vi "Autonomous Independent.vi"() -> ()   [LabVIEW 2016]
doc: "This VI is called when autonomous begins, and will automatically be terminated when autonomous ends. You can carry out timed or sensor driven robot movement independently without needing to return to the caller."
uses:
  2_8_17/Auto_Action.ctl
  <vilib>/Rock Robotics/Network Tables/NT Read Number.vi
  2_11_17/Systems/Global 1.vi
panel:
  out "Auto Mode":dbl=10.0
  in  "Auton_Modes":T2(array[cluster])=[{"Actions"=[{"Effort"=0.55, "Duration"=3.5, "Action"=enum."Nothing", "Encoder"=0.0, "Condition"=FALSE}, {"Effort"=0.0, "Duration"=0.0, "Action"=enum."Nothing", "Encoder"=0.0, "Condition"=FALSE}]}, {"Actions"=[{"Effort"=0.53, "Duration"=1.0, "Action"=enum."Shoot", "Encoder"=6.462, "Condition"=TRUE}, {"Effort"=0.0, "Duration"=3.0, "Action"=enum."Index", "Encoder"=0.0, "Condition"=FALSE}, {"Effort"=0.3, "Duration"=2.0, "Action"=enum."Turn", "Encoder"=38.0, "Condition"=FALSE}, {"Effort"=0.3, "Duration"=5.0, "Action"=enum."Drive", "Encoder"=0.0, "Condition"=TRUE}, {"Effort"=0.25, "Duration"=0.0, "Action"=enum."Nothing", "Encoder"=57.0, "Condition"=FALSE}, {"Effort"=-0.25, "Duration"=0.0, "Action"=enum."Nothing", "Encoder"=0.0, "Condition"=FALSE}, {"Effort"=1.0, "Duration"=0.0, "Action"=enum."Nothing", "Encoder"=0.0, "Condition"=FALSE}, {"Effort"=0.25, "Duration"=0.0, "Action"=enum."Nothing", "Encoder"=0.0, "Condition"=FALSE}]}, {"Actions"=[{"Effort"=0.0, "Duration"=0.1, "Action"=enum."Drive Encoder Reset", "Encoder"=0.0, "Condition"=FALSE}, {"Effort"=0.0, "Duration"=1.0, "Action"=enum."Gyro Reset", "Encoder"=0.0, "Condition"=FALSE}, {"Effort"=0.3, "Duration"=2.5, "Action"=enum."Drive", "Encoder"=1000.0, "Condition"=TRUE}, {"Effort"=1.0, "Duration"=1.0, "Action"=enum."Gear0", "Encoder"=0.0, "Condition"=FALSE}, {"Effort"=1.0, "Duration"=0.0, "Action"=enum."Nothing", "Encoder"=0.0, "Condition"=FALSE}, {"Effort"=1.0, "Duration"=0.5, "Action"=enum."Nothing", "Encoder"=0.0, "Condition"=FALSE}, {"Effort"=0.0, "Duration"=0.0, "Action"=enum."Drive Encoder Reset", "Encoder"=0.0, "Condition"=FALSE}, {"Effort"=0.3, "Duration"=0.5, "Action"=enum."Nothing", "Encoder"=24.0, "Condition"=TRUE}, {"Effort"=0.0, "Duration"=0.0, "Action"=enum."Nothing", "Encoder"=0.0, "Condition"=FALSE}, {"Effort"=-0.2, "Duration"=2.0, "Action"=enum."Drive", "Encoder"=24.0, "Condition"=TRUE}, {"Effort"=0.0, "Duration"=0.0, "Action"=enum."Drive Encoder Reset", "Encoder"=0.0, "Condition"=FALSE}, {"Effort"=-0.25, "Duration"=0.0, "Action"=enum."Nothing", "Encoder"=12.0, "Condition"=FALSE}]}, {"Actions"=[{"Effort"=0.0, "Duration"=0.1, "Action"=enum."Drive Encoder Reset", "Encoder"=6.462, "Condition"=FALSE}, {"Effort"=0.0, "Duration"=0.1, "Action"=enum."Gyro Reset", "Encoder"=0.0, "Condition"=FALSE}, {"Effort"=-0.25, "Duration"=1.0, "Action"=enum."Drive", "Encoder"=6.462, "Condition"=FALSE}, {"Effort"=0.0, "Duration"=0.1, "Action"=enum."Gyro Reset", "Encoder"=0.0, "Condition"=FALSE}, {"Effort"=-0.25, "Duration"=0.0, "Action"=enum."Turn", "Encoder"=0.0, "Condition"=FALSE}, {"Effort"=-0.25, "Duration"=0.0, "Action"=enum."Drive", "Encoder"=7.5, "Condition"=FALSE}, {"Effort"=-1.0, "Duration"=0.0, "Action"=enum."Gear0", "Encoder"=0.0, "Condition"=FALSE}, {"Effort"=0.25, "Duration"=0.0, "Action"=enum."Drive", "Encoder"=3.0, "Condition"=FALSE}]}, {"Actions"=[{"Effort"=0.0, "Duration"=0.1, "Action"=enum."Drive Encoder Reset", "Encoder"=6.462, "Condition"=FALSE}, {"Effort"=0.0, "Duration"=0.1, "Action"=enum."Gyro Reset", "Encoder"=0.0, "Condition"=FALSE}, {"Effort"=-0.25, "Duration"=1.0, "Action"=enum."Drive", "Encoder"=6.462, "Condition"=FALSE}, {"Effort"=0.0, "Duration"=0.1, "Action"=enum."Gyro Reset", "Encoder"=0.0, "Condition"=FALSE}, {"Effort"=-0.25, "Duration"=0.0, "Action"=enum."Turn", "Encoder"=0.0, "Condition"=FALSE}, {"Effort"=-0.25, "Duration"=0.0, "Action"=enum."Drive", "Encoder"=7.5, "Condition"=FALSE}, {"Effort"=-1.0, "Duration"=0.0, "Action"=enum."Gear0", "Encoder"=0.0, "Condition"=FALSE}, {"Effort"=0.25, "Duration"=0.0, "Action"=enum."Drive", "Encoder"=3.0, "Condition"=FALSE}]}, {"Actions"=[{"Effort"=0.0, "Duration"=0.1, "Action"=enum."Drive Encoder Reset", "Encoder"=0.0, "Condition"=FALSE}, {"Effort"=0.0, "Duration"=0.1, "Action"=enum."Gyro Reset", "Encoder"=0.0, "Condition"=FALSE}, {"Effort"=0.25, "Duration"=1.0, "Action"=enum."Drive", "Encoder"=6.462, "Condition"=FALSE}, {"Effort"=1.0, "Duration"=0.1, "Action"=enum."Gyro Reset", "Encoder"=0.0, "Condition"=FALSE}, {"Effort"=0.25, "Duration"=0.0, "Action"=enum."Turn", "Encoder"=0.0, "Condition"=FALSE}, {"Effort"=0.25, "Duration"=0.0, "Action"=enum."Drive", "Encoder"=7.5, "Condition"=FALSE}, {"Effort"=1.0, "Duration"=0.0, "Action"=enum."Gear0", "Encoder"=0.0, "Condition"=FALSE}, {"Effort"=-0.25, "Duration"=0.0, "Action"=enum."Drive", "Encoder"=3.0, "Condition"=FALSE}]}, {"Actions"=[{"Effort"=0.0, "Duration"=0.1, "Action"=enum."Nothing", "Encoder"=0.0, "Condition"=FALSE}, {"Effort"=0.0, "Duration"=0.1, "Action"=enum."Gyro Reset", "Encoder"=0.0, "Condition"=FALSE}, {"Effort"=0.25, "Duration"=5.0, "Action"=enum."Drive", "Encoder"=60000.0, "Condition"=TRUE}, {"Effort"=0.75, "Duration"=1.0, "Action"=enum."Nothing", "Encoder"=0.0, "Condition"=FALSE}, {"Effort"=0.0, "Duration"=1.0, "Action"=enum."Nothing", "Encoder"=0.0, "Condition"=FALSE}, {"Effort"=0.0, "Duration"=0.0, "Action"=enum."Nothing", "Encoder"=0.0, "Condition"=FALSE}]}, {"Actions"=[{"Effort"=0.0, "Duration"=0.5, "Action"=enum."Drive Encoder Reset", "Encoder"=0.0, "Condition"=FALSE}, {"Effort"=0.55, "Duration"=4.25, "Action"=enum."Gyro Reset", "Encoder"=0.0, "Condition"=FALSE}, {"Effort"=-0.5, "Duration"=0.0, "Action"=enum."Drive", "Encoder"=46.0, "Condition"=FALSE}, {"Effort"=0.3, "Duration"=1.0, "Action"=enum."Nothing", "Encoder"=0.0, "Condition"=FALSE}, {"Effort"=0.3, "Duration"=2.0, "Action"=enum."Vision Correction", "Encoder"=76.6, "Condition"=FALSE}, {"Effort"=-0.25, "Duration"=1.0, "Action"=enum."Drive", "Encoder"=18.5, "Condition"=TRUE}, {"Effort"=1.0, "Duration"=0.0, "Action"=enum."Gear0", "Encoder"=0.0, "Condition"=FALSE}, {"Effort"=0.3, "Duration"=1.3, "Action"=enum."Drive", "Encoder"=30.0, "Condition"=TRUE}, {"Effort"=0.0, "Duration"=0.0, "Action"=enum."Nothing", "Encoder"=0.0, "Condition"=FALSE}, {"Effort"=0.03, "Duration"=0.0, "Action"=enum."Turn", "Encoder"=0.0, "Condition"=FALSE}, {"Effort"=0.0, "Duration"=0.0, "Action"=enum."Drive", "Encoder"=0.0, "Condition"=FALSE}]}, {"Actions"=[{"Effort"=0.0, "Duration"=0.0, "Action"=enum."Nothing", "Encoder"=0.0, "Condition"=FALSE}]}, {"Actions"=[{"Effort"=0.0, "Duration"=2.5, "Action"=enum."Shoot", "Encoder"=0.0, "Condition"=FALSE}, {"Effort"=0.0, "Duration"=5.0, "Action"=enum."Index", "Encoder"=0.0, "Condition"=FALSE}, {"Effort"=0.25, "Duration"=3.5, "Action"=enum."Nothing", "Encoder"=88.0, "Condition"=FALSE}, {"Effort"=1.0, "Duration"=1.0, "Action"=enum."Nothing", "Encoder"=0.0, "Condition"=FALSE}, {"Effort"=1.0, "Duration"=1.0, "Action"=enum."Nothing", "Encoder"=0.0, "Condition"=FALSE}, {"Effort"=1.0, "Duration"=0.5, "Action"=enum."Nothing", "Encoder"=0.0, "Condition"=FALSE}, {"Effort"=0.0, "Duration"=0.0, "Action"=enum."Nothing", "Encoder"=0.0, "Condition"=FALSE}, {"Effort"=-0.25, "Duration"=0.0, "Action"=enum."Nothing", "Encoder"=3.0, "Condition"=FALSE}, {"Effort"=0.0, "Duration"=0.0, "Action"=enum."Nothing", "Encoder"=0.0, "Condition"=FALSE}, {"Effort"=0.25, "Duration"=0.0, "Action"=enum."Nothing", "Encoder"=24.0, "Condition"=FALSE}, {"Effort"=0.0, "Duration"=0.0, "Action"=enum."Nothing", "Encoder"=0.0, "Condition"=FALSE}, {"Effort"=-0.25, "Duration"=0.0, "Action"=enum."Nothing", "Encoder"=12.0, "Condition"=FALSE}]}, {"Actions"=[{"Effort"=0.0, "Duration"=0.1, "Action"=enum."Drive Encoder Reset", "Encoder"=0.0, "Condition"=FALSE}, {"Effort"=0.0, "Duration"=1.0, "Action"=enum."Gyro Reset", "Encoder"=0.0, "Condition"=FALSE}, {"Effort"=0.3, "Duration"=1.4, "Action"=enum."Drive", "Encoder"=88.0, "Condition"=TRUE}, {"Effort"=0.3, "Duration"=4.0, "Action"=enum."Turn", "Encoder"=2.0, "Condition"=TRUE}, {"Effort"=1.0, "Duration"=1.0, "Action"=enum."Nothing", "Encoder"=0.0, "Condition"=FALSE}, {"Effort"=1.0, "Duration"=0.5, "Action"=enum."Nothing", "Encoder"=0.0, "Condition"=FALSE}, {"Effort"=0.0, "Duration"=0.0, "Action"=enum."Nothing", "Encoder"=0.0, "Condition"=FALSE}, {"Effort"=-0.25, "Duration"=0.0, "Action"=enum."Nothing", "Encoder"=3.0, "Condition"=FALSE}, {"Effort"=0.0, "Duration"=0.0, "Action"=enum."Nothing", "Encoder"=0.0, "Condition"=FALSE}, {"Effort"=0.25, "Duration"=0.0, "Action"=enum."Nothing", "Encoder"=24.0, "Condition"=FALSE}, {"Effort"=0.0, "Duration"=0.0, "Action"=enum."Nothing", "Encoder"=0.0, "Condition"=FALSE}, {"Effort"=-0.25, "Duration"=0.0, "Action"=enum."Nothing", "Encoder"=12.0, "Condition"=FALSE}]}, {"Actions"=[{"Effort"=0.0, "Duration"=1.0, "Action"=enum."Drive Encoder Reset", "Encoder"=0.0, "Condition"=FALSE}, {"Effort"=0.0, "Duration"=1.0, "Action"=enum."Shoot", "Encoder"=0.0, "Condition"=FALSE}, {"Effort"=0.25, "Duration"=5.0, "Action"=enum."Index", "Encoder"=88.0, "Condition"=FALSE}, {"Effort"=1.0, "Duration"=1.0, "Action"=enum."Nothing", "Encoder"=0.0, "Condition"=FALSE}, {"Effort"=1.0, "Duration"=1.0, "Action"=enum."Nothing", "Encoder"=0.0, "Condition"=FALSE}, {"Effort"=1.0, "Duration"=0.5, "Action"=enum."Nothing", "Encoder"=0.0, "Condition"=FALSE}, {"Effort"=0.0, "Duration"=0.0, "Action"=enum."Nothing", "Encoder"=0.0, "Condition"=FALSE}, {"Effort"=-0.25, "Duration"=0.0, "Action"=enum."Nothing", "Encoder"=3.0, "Condition"=FALSE}, {"Effort"=0.0, "Duration"=0.0, "Action"=enum."Nothing", "Encoder"=0.0, "Condition"=FALSE}, {"Effort"=0.25, "Duration"=0.0, "Action"=enum."Nothing", "Encoder"=24.0, "Condition"=FALSE}, {"Effort"=0.0, "Duration"=0.0, "Action"=enum."Nothing", "Encoder"=0.0, "Condition"=FALSE}, {"Effort"=-0.25, "Duration"=0.0, "Action"=enum."Nothing", "Encoder"=12.0, "Condition"=FALSE}]}, {"Actions"=[{"Effort"=0.0, "Duration"=0.1, "Action"=enum."Drive Encoder Reset", "Encoder"=0.0, "Condition"=FALSE}, {"Effort"=0.0, "Duration"=1.0, "Action"=enum."Gyro Reset", "Encoder"=0.0, "Condition"=FALSE}, {"Effort"=0.3, "Duration"=1.4, "Action"=enum."Drive", "Encoder"=88.0, "Condition"=TRUE}, {"Effort"=0.3, "Duration"=4.0, "Action"=enum."Turn", "Encoder"=0.0, "Condition"=TRUE}, {"Effort"=1.0, "Duration"=1.0, "Action"=enum."Nothing", "Encoder"=0.0, "Condition"=FALSE}, {"Effort"=1.0, "Duration"=0.5, "Action"=enum."Nothing", "Encoder"=0.0, "Condition"=FALSE}, {"Effort"=0.0, "Duration"=0.0, "Action"=enum."Nothing", "Encoder"=0.0, "Condition"=FALSE}, {"Effort"=0.3, "Duration"=0.5, "Action"=enum."Nothing", "Encoder"=24.0, "Condition"=TRUE}, {"Effort"=0.0, "Duration"=0.0, "Action"=enum."Nothing", "Encoder"=0.0, "Condition"=FALSE}, {"Effort"=-0.2, "Duration"=2.0, "Action"=enum."Nothing", "Encoder"=24.0, "Condition"=TRUE}, {"Effort"=0.0, "Duration"=0.0, "Action"=enum."Nothing", "Encoder"=0.0, "Condition"=FALSE}, {"Effort"=-0.25, "Duration"=0.0, "Action"=enum."Nothing", "Encoder"=12.0, "Condition"=FALSE}]}]
  # "Nothing"
  # "Boiler Right Right side gear"
  # "Middle Gear"
  # "Boiler Right Left Side Gear"
  # "Boiler Left RightSide Gear"
  # "Boiler Left Left Side Gear"
  # "Drive"
  # "Vision Correction"
  # "Hopper"
  # "10 ball"
  # "Farside"
  # "Boilerside-10 ball"
  # "Auto 5"
  # "Auto 6"
  # "Auto 6"
  # "Auto 7"
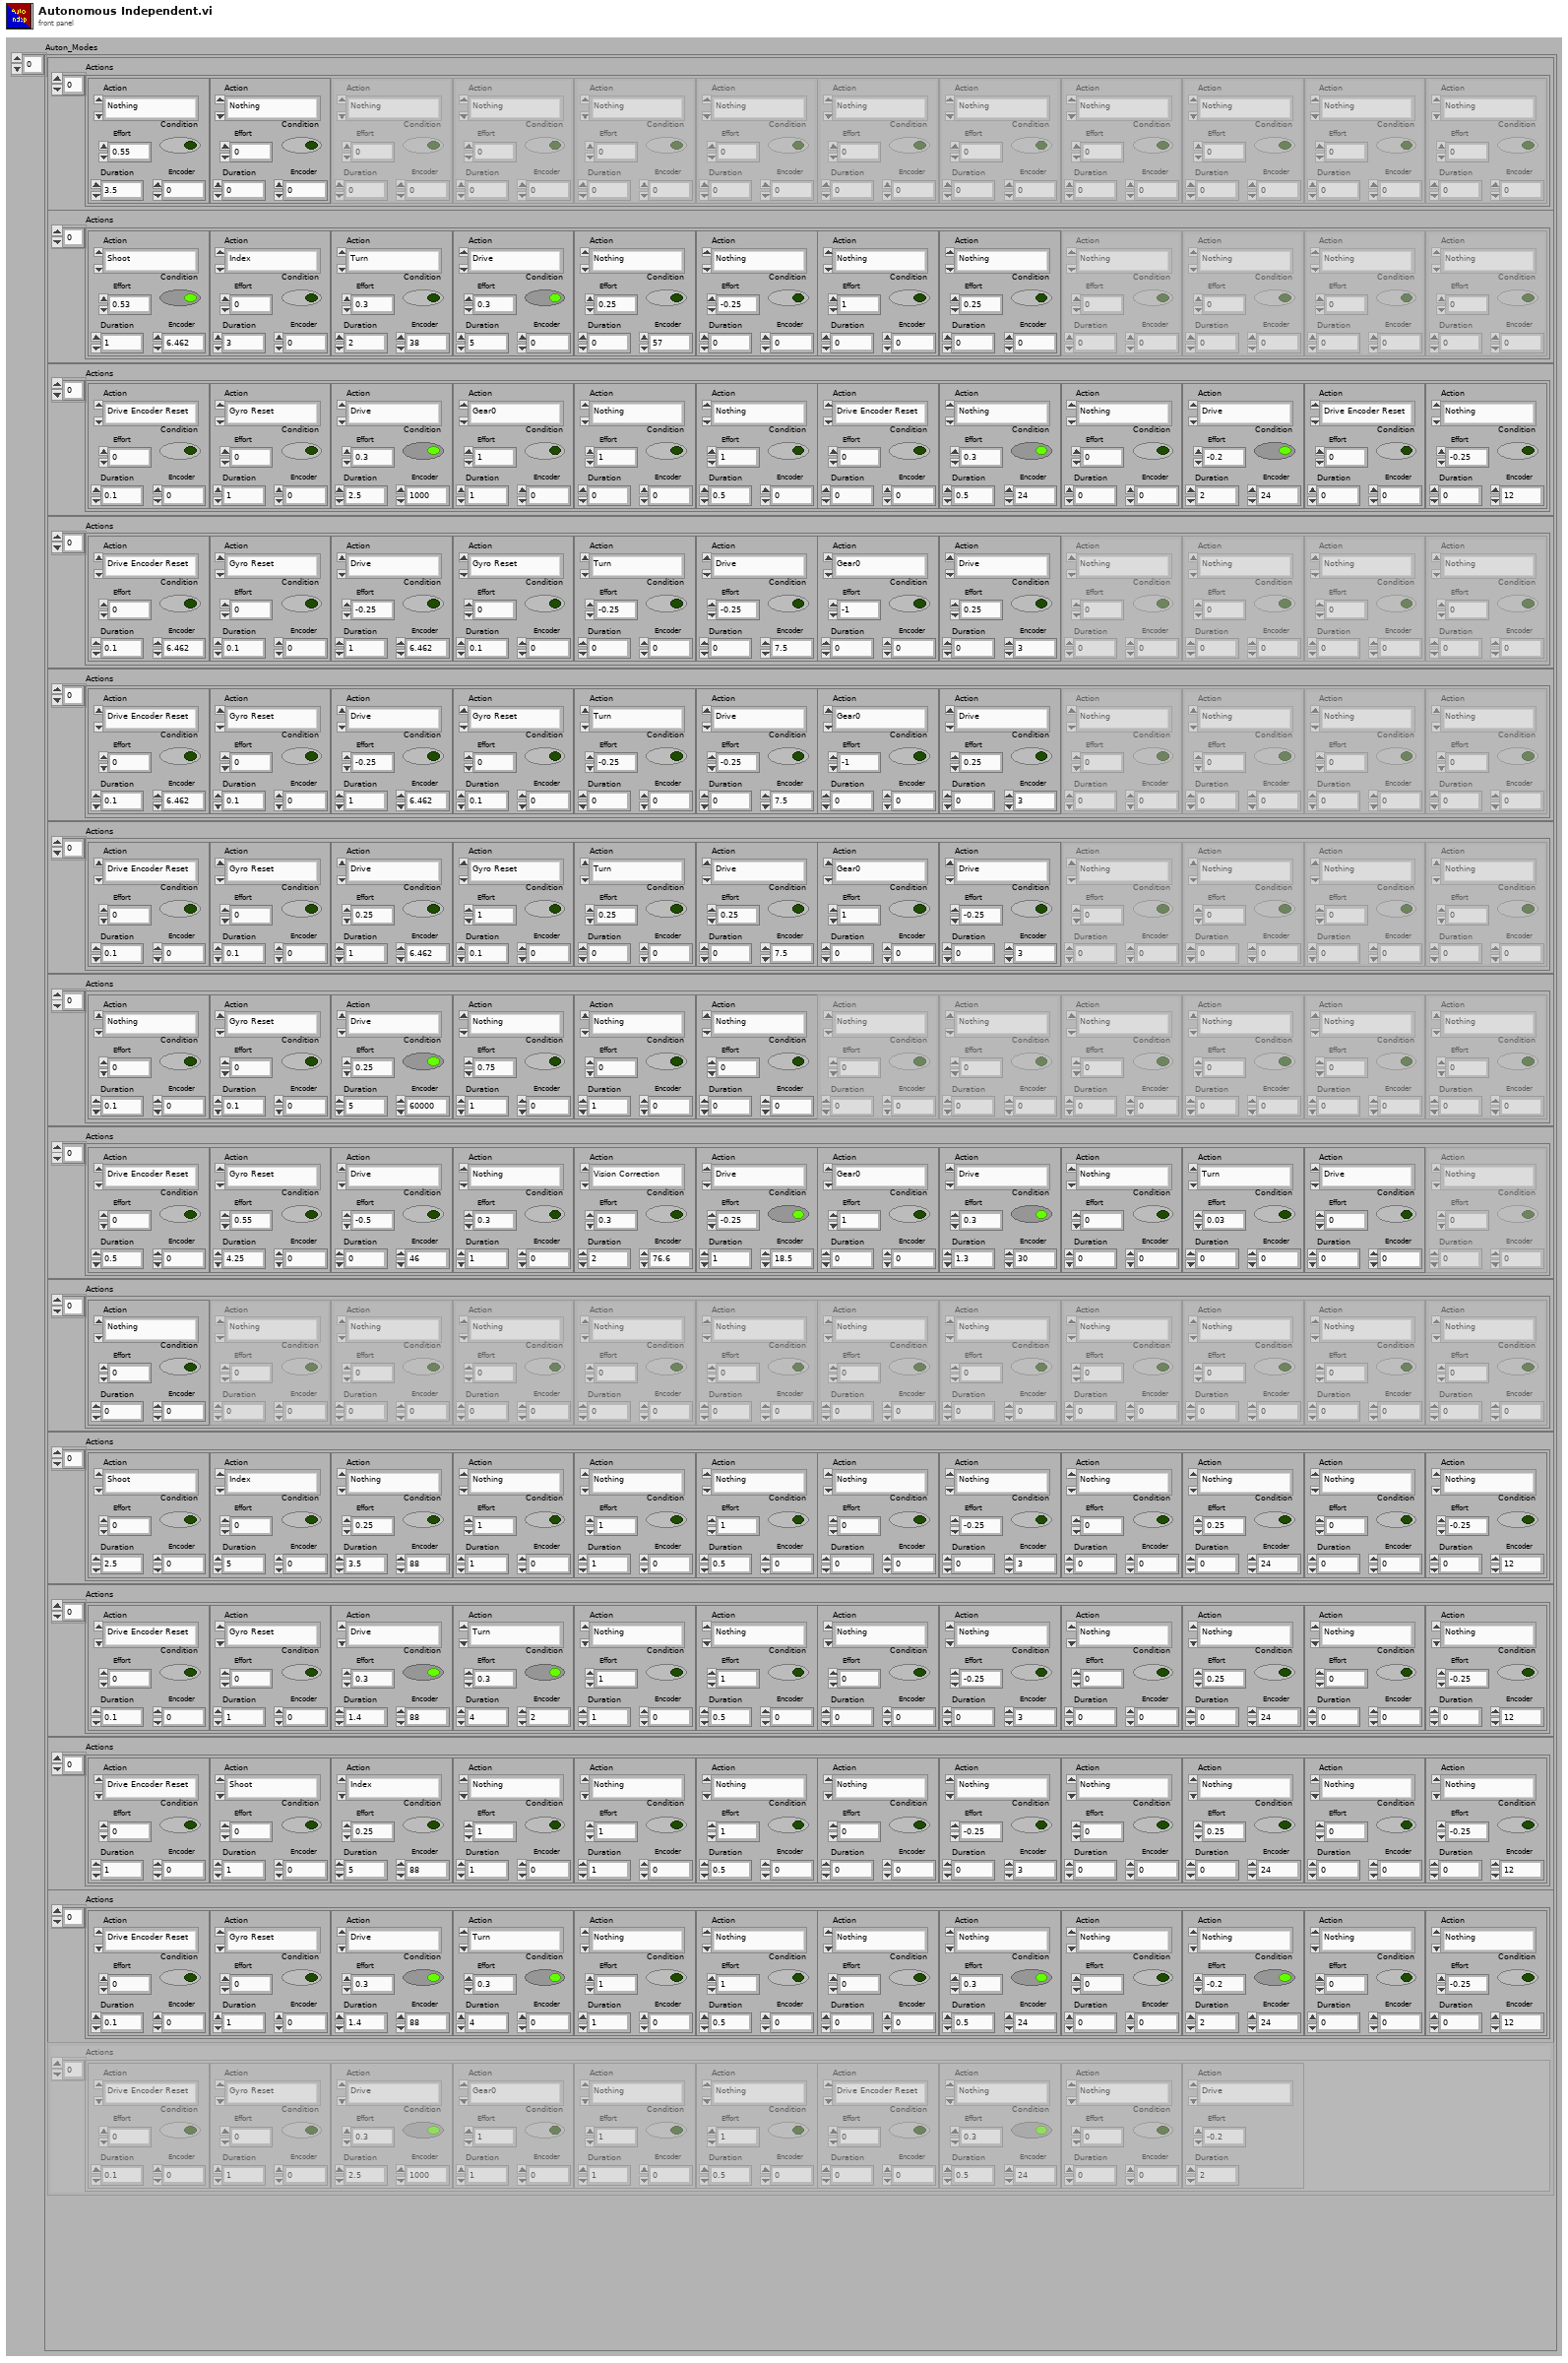
[diagram p1: front panel]
types:
  T1 = typedef "Auto_Action.ctl" = enum16{"Nothing", "Drive", "Vision Correction", "Turn", "Gear0", "Gear1", "Climb", "Intake", "Index", "Shoot", "Test", "Drive Encoder Reset", "Gyro Reset"}
  T2 = cluster{"Actions":cluster{"Effort":dbl, "Duration":dbl, "Action":T1, "Encoder":dbl, "Condition":bool}[]}[]
  T3 = cluster{"Actions":cluster{"Effort":dbl, "Duration":dbl, "Action":T1, "Encoder":dbl, "Condition":bool}[]}
  T4 = cluster{"Effort":dbl, "Duration":dbl, "Action":T1, "Encoder":dbl, "Condition":bool}[]
  T5 = typedef "WPI_MotorControlDeviceRef.ctl" = cluster{"DeviceStatus":errorcluster, "Type":T6, "PWM":cluster{"PWM Channel":T7, "DeadBand":T8}, "CAN":cluster{"Device Number":u8, "SetOutput VI Ref":variant, "GetOutput VI Ref":variant, "Enable VI Ref":variant, "Disable VI Ref":variant, "Data":variant}, "Invert":bool}
  T6 = typedef "WPI_MotorControlType.ctl" = enum16{"PWM", "CAN"}
  T7 = typedef "FPGA_DIOPWMChannel.ctl" = enum8{"PWM 0", "PWM 1", "PWM 2", "PWM 3", "PWM 4", "PWM 5", "PWM 6", "PWM 7", "PWM 8", "PWM 9", "PWM MXP 0", "PWM MXP 1", "PWM MXP 2", "PWM MXP 3", "PWM MXP 4", "PWM MXP 5", "PWM MXP 6", "PWM MXP 7", "PWM MXP 8", "PWM MXP 9", "Invalid"}
  T8 = typedef "WPI_PWMDeadband.ctl" = cluster{"Name":string, "maxPositivePwm":i32, "minPositivePwm":i32, "centerPwm":i32, "maxNegativePwm":i32, "minNegativePwm":i32, "angularRange":u16}
  T9 = typedef "WPI_CANTalonSRX_GlobalStatus.ctl" = cluster{"Applied Throttle":dbl, "Module Enabled":bool, "CAN Error":errorcluster, "Closed Loop Error":dbl, "Forward Limit Switch Closed":bool, "Reverse Limit Switch Closed":bool, "Sensor Position":dbl, "Sensor Velocity":dbl, "Current":dbl, "Sticky Fault - Over Temp":bool, "Sticky Fault - Under Voltage":bool, "Sticky Fault - Forward Limit":bool, "Sticky Fault - Reverse Limit":bool, "Sticky Fault - Forward Soft Limit":bool, "Sticky Fault - Reverse Soft Limit":bool, "Brake is Enabled":bool, "Encoder Position":dbl, "Encoder Velocity":dbl, "Encoder Index Count":dbl, "Encoder A Pin State":bool, "Encoder B Pin State":bool, "Encoder Index Pin State":bool, "Analog In":dbl, "Analog In Velocity":dbl, "Temperature (C)":dbl, "Battery Voltage":dbl, "Control 5 Is Supported":bool, "Current Profile Slot Select":dbl, "Pos Div 8":bool, "Vel Div 4":bool, "Pulse Width Position":i32, "Pulse Width Velocity":i32, "Pulse Width Rise To Rise (us)":i32, "Pulse Width Rise To Fall (us)":i32, "Mot Prof Active Is Under Run":bool, "Mot Prof Active Has Under Run":bool, "Mot Prof Active Is Last":bool, "Mot Prof Active Velocity Only":bool, "Mot Prof Active Is Valid":bool, "Mot Prof Buffer Is Full":bool, "Mot Prof Active Profile Slot Select":i32, "Mot Prof NextID":i32, "Mot Prof Count":i32, "Mot Prof Active Velocity":dbl, "Mot Prof Active Position":dbl, "Mot Prof Output Enable":i32}
  T10 = typedef "WPI_GyroDevRef.ctl" = cluster{"DevStatus":errorcluster, "Analog Channel":T11, "Offset":dbl, "Gain (VoltsPerDegree/Second)":dbl, "Gyro Type":enum16{"Analog", "XRS450"}, "Handle":i32, "SPI Bus":T12, "Device Found":bool, "Sample Rate":dbl, "Calibrate On Open":bool}
  T11 = typedef "FPGA_AIChannel.ctl" = enum8{"AI 0", "AI 1", "AI 2", "AI 3", "AI MXP 0", "AI MXP 1", "AI MXP 2", "AI MXP 3", "Invalid"}
  T12 = typedef "spi_bus.ctl" = enum16{"SPI On-Board, CS0", "SPI On-Board, CS1", "SPI On-Board, CS2", "SPI On-Board, CS3", "SPI MXP", "Invalid"}
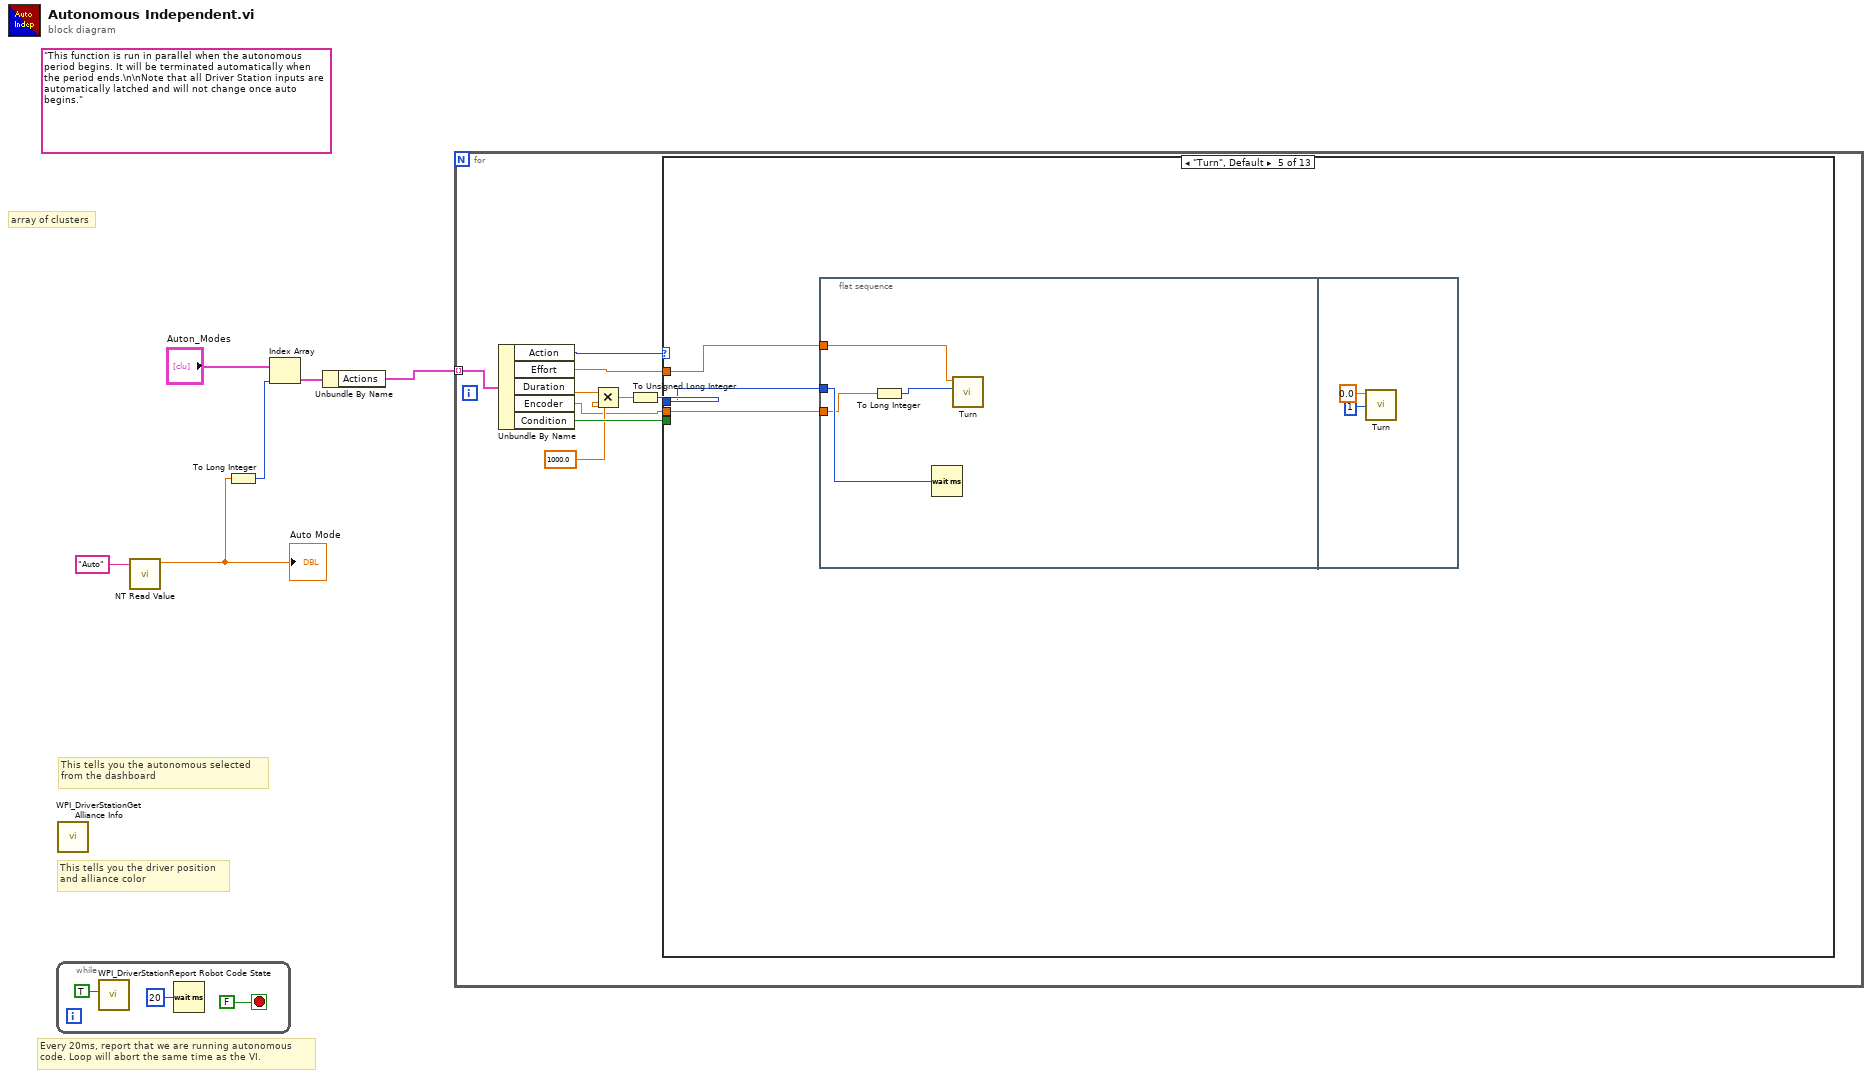
[diagram p0: block diagram]
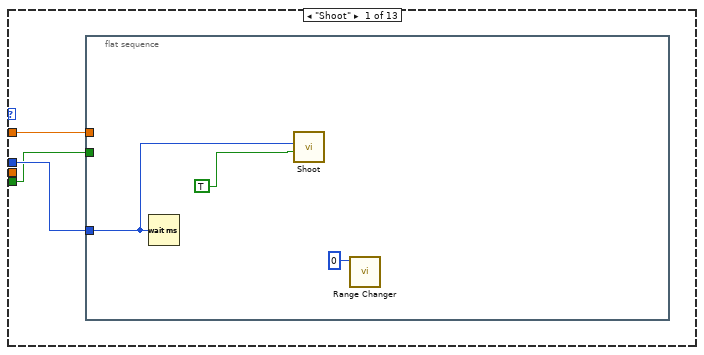
[diagram p2: hidden frame]
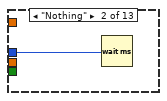
[diagram p3: hidden frame]
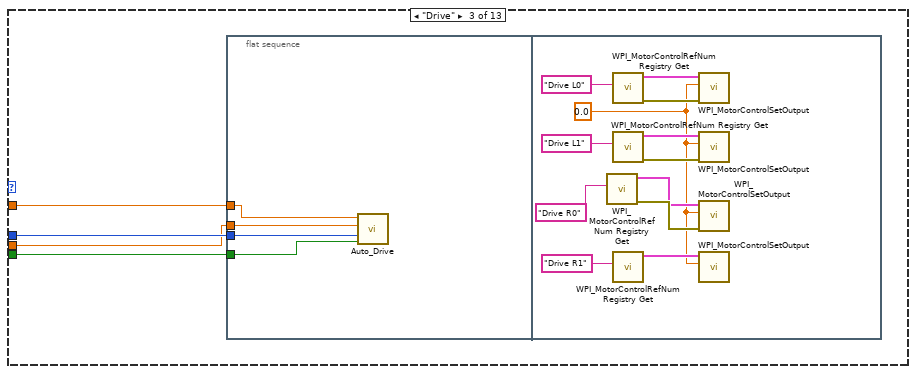
[diagram p4: hidden frame]
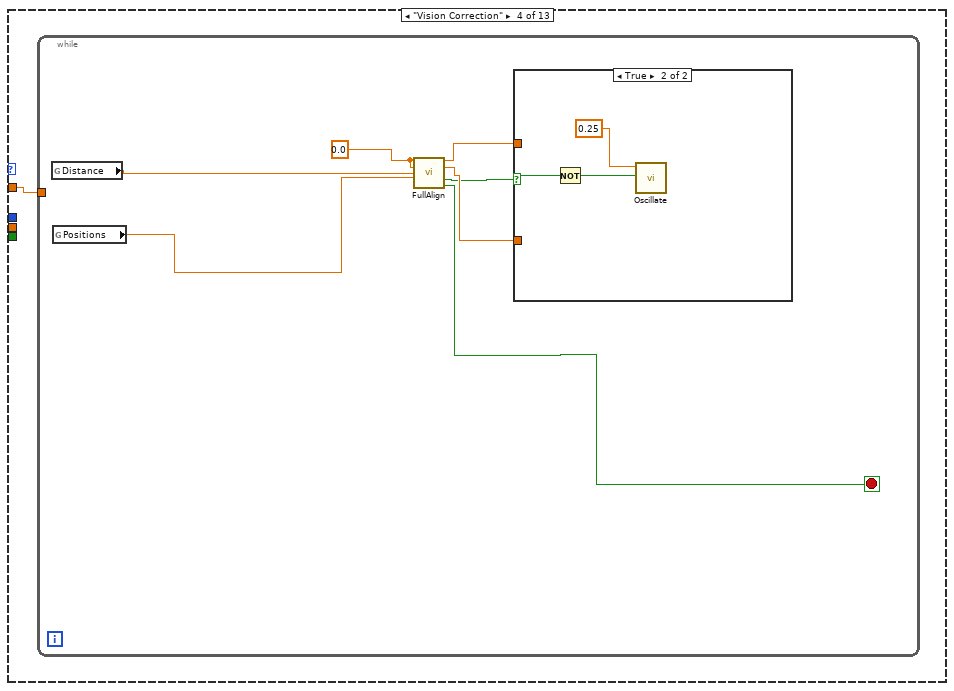
[diagram p5: hidden frame]
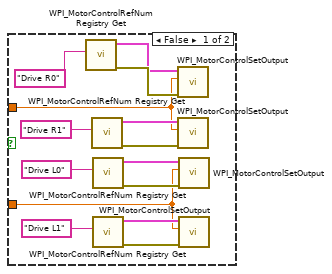
[diagram p6: hidden frame]
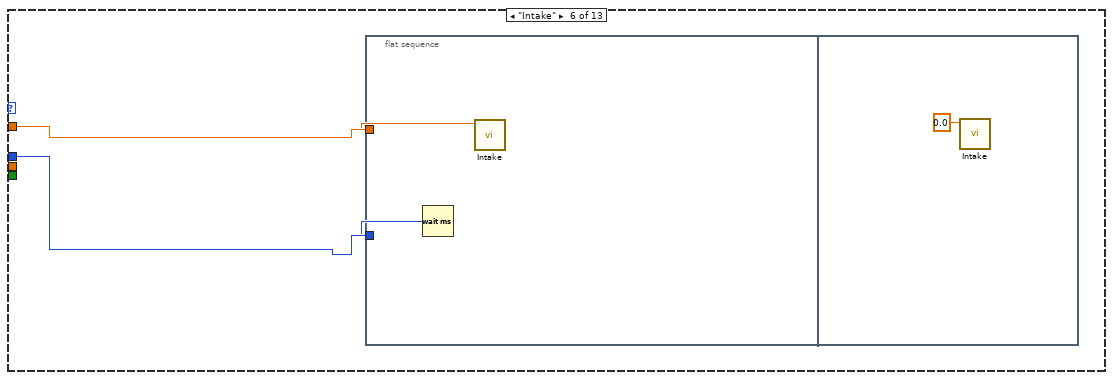
[diagram p7: hidden frame]
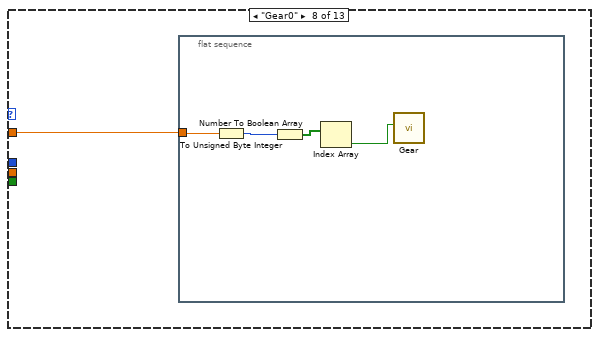
[diagram p9: hidden frame]
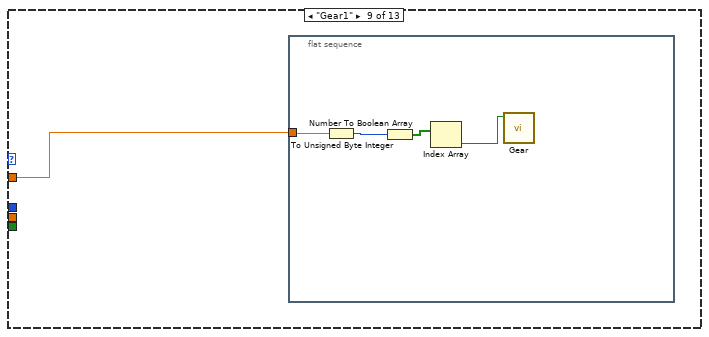
[diagram p10: hidden frame]
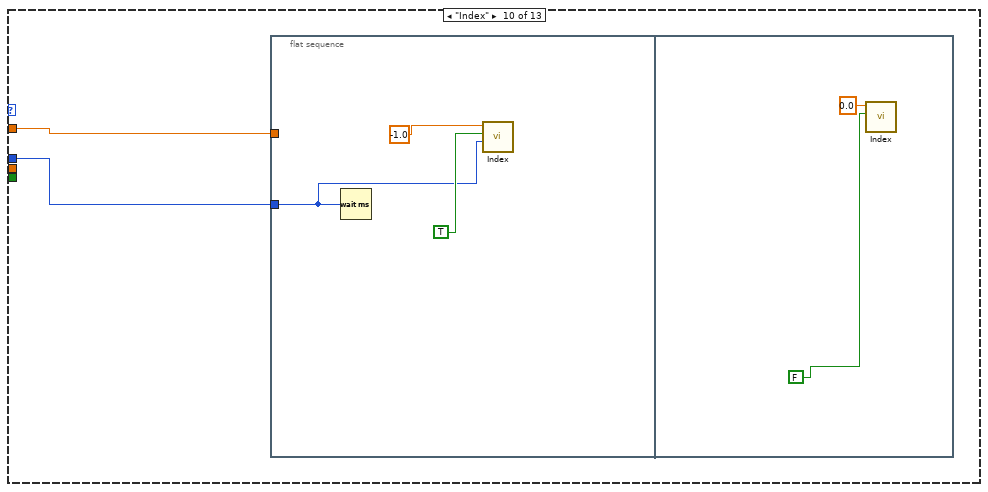
[diagram p11: hidden frame]
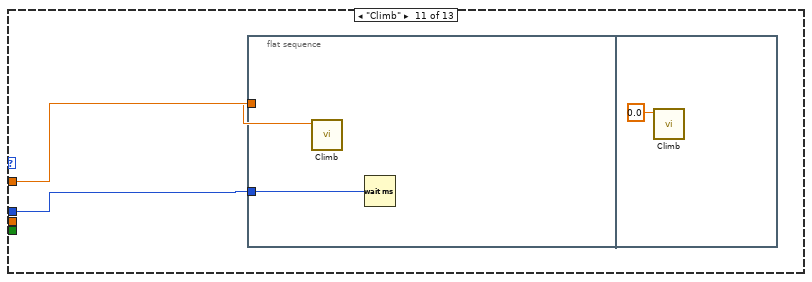
[diagram p12: hidden frame]
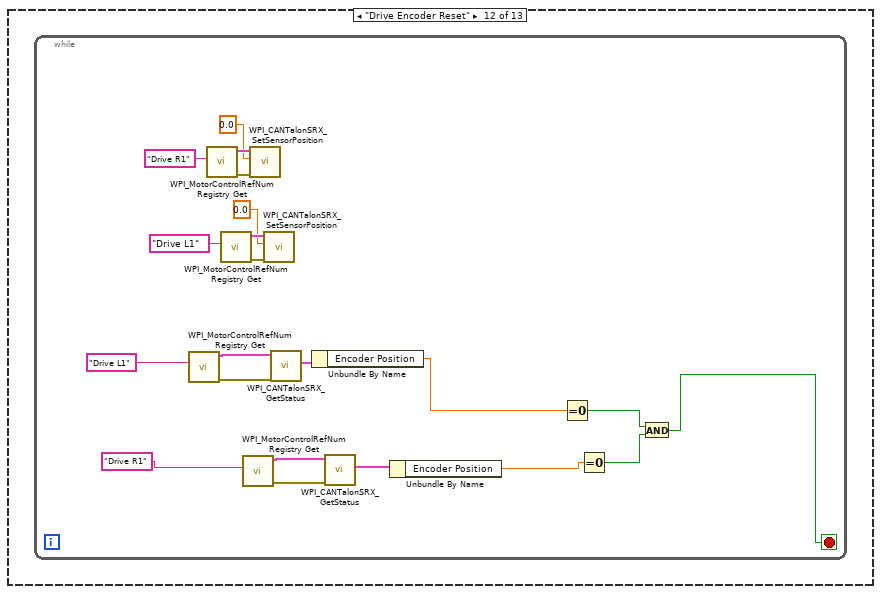
[diagram p13: hidden frame]
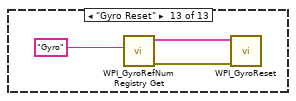
[diagram p14: hidden frame]
diagram:
  (unwired) "This function is run in parallel when the autonomous period begins. It will be terminated automatically when the period ends.\n\nNote that all Driver Station inputs are automatically latched and will not change once auto begins."
  # "This tells you the autonomous selected\nfrom the dashboard"
  # "array of clusters"
  # "Every 20ms, report that we are running autonomous\ncode. Loop will abort the same time as the VI."
  # "This tells you the driver position\nand alliance color"
  n1 = while {
    stop <- FALSE stop-if-true
    n2 = call <vilib>:"WPI_DriverStationReport Robot Code State.vi"("Autonomous"=TRUE) -> ()  [unwired: 10 in, 1 out]
    n3 = Wait (ms)(milliseconds to wait=u32 20) -> ()  [unwired: 1 out]
  }
  n4 = call <vilib>:"WPI_DriverStationGet Alliance Info.vi"() -> ()  [unwired: 12 out]
  n5 = call-poly <vilib>:"NT Read Value.vi"("Name"="Auto") -> ("Numeric"=w1:dbl)  [unwired: 9 in, 1 out]
  "Auto Mode" <- w1
  n6 = To Long Integer(number=w1) -> (32bit integer=w3:i32)
  n7 = Index Array(array="Auton_Modes", index=w3) -> (element=w5:T3)
  n8 = Unbundle By Name(w5) -> ("Actions"=w6:T4)
  n9 = for {
    tunnel: w6 -> [w18] mode=indexing
    n10 = Unbundle By Name(w18) -> ("Action"=w17:T1, "Effort"=w16:dbl, "Duration"=w15:dbl, "Encoder"=w10:dbl, "Condition"=w12:bool)
    n11 = Multiply(x=w15, y=1000.0) -> (x*y=w14:dbl)
    n12 = To Unsigned Long Integer(number=w14) -> (unsigned 32bit integer=w13:u32)
    n13 = case shown="\"Turn\", Default" w17 {
      tunnel: w16 -> [w21 _ w29 w46 w73 w81 _ w85 w90 w95 w103 _ _]
      tunnel: w13 -> [w20 w25 w28 _ w72 w80 _ _ _ w96 w102 _ _]
      tunnel: w12 -> [w19 _ w27 _ _ _ _ _ _ _ _ _ _]
      tunnel: w10 -> [_ _ w26 _ w71 _ _ _ _ _ _ _ _]
      frame "Shoot" {
        n14 = flat-sequence {
          tunnel: w21 -> [_]
          tunnel: w20 -> [w22]
          tunnel: w19 -> [_]
          frame #0 {
            n15 = Wait (ms)(milliseconds to wait=w22) -> ()  [unwired: 1 out]
            n16 = call "Shoot.vi"("millisecond timer value"=w22, "Shoot"=TRUE) -> ()  [unwired: 9 in]
            n17 = call "Range Changer.vi"("POV"=i16 0) -> ()  [unwired: 10 in, 1 out]
          }
        }
      }
      frame "Nothing" {
        n18 = Wait (ms)(milliseconds to wait=w25) -> ()  [unwired: 1 out]
      }
      frame "Drive" {
        n19 = flat-sequence {
          tunnel: w29 -> [w33]
          tunnel: w28 -> [w32]
          tunnel: w27 -> [w31]
          tunnel: w26 -> [w30]
          frame #0 {
            n20 = call "Auto_Drive.vi"("Timer?"=w31, "Duration"=w32, "distance"=w30, "Drive Effort"=w33) -> ()  [unwired: 8 in]
          }
          frame #1 {
            w34 = 0.0 ("Drive L")
            n21 = call <vilib>:"WPI_MotorControlRefNum Registry Get.vi"("refnum name"="Drive R0") -> ("error out"=w39:errorcluster, "MotorControlDevRef"=w35:T5)  [unwired: 9 in]
            n22 = call <vilib>:"WPI_MotorControlRefNum Registry Get.vi"("refnum name"="Drive L0") -> ("error out"=w40:errorcluster, "MotorControlDevRef"=w41:T5)  [unwired: 9 in]
            n23 = call <vilib>:"WPI_MotorControlRefNum Registry Get.vi"("refnum name"="Drive L1") -> ("error out"=w44:errorcluster, "MotorControlDevRef"=w43:T5)  [unwired: 9 in]
            n24 = call <vilib>:"WPI_MotorControlRefNum Registry Get.vi"("refnum name"="Drive R1") -> ("MotorControlDevRef"=w37:T5)  [unwired: 9 in, 1 out]
            n25 = call <vilib>:"WPI_MotorControlSetOutput.vi"("error in (no error)"=w40, "Output"=w34, "MotorControlDevRef"=w41) -> ()  [unwired: 6 in, 3 out]
            n26 = call <vilib>:"WPI_MotorControlSetOutput.vi"("error in (no error)"=w44, "Output"=w34, "MotorControlDevRef"=w43) -> ()  [unwired: 6 in, 3 out]
            n27 = call <vilib>:"WPI_MotorControlSetOutput.vi"("error in (no error)"=w39, "Output"=w34, "MotorControlDevRef"=w35) -> ()  [unwired: 6 in, 3 out]
            n28 = call <vilib>:"WPI_MotorControlSetOutput.vi"("Output"=w34, "MotorControlDevRef"=w37) -> ()  [unwired: 7 in, 3 out]
          }
        }
      }
      frame "Vision Correction" {
        n29 = while {
          tunnel: w46 -> [_]
          stop <- w48 stop-if-true
          w51 = 0.0
          n30 = global read "Global 1.vi" "Distance"() -> (w50:dbl)
          n31 = global read "Global 1.vi" "Positions"() -> (w49:dbl)
          n32 = call "FullAlign.vi"("Joystick 0"=w51, "Joystick 1"=w51, "Distance"=w50, "Angle"=w49) -> ("Right Motor"=w53:dbl, "Left Motor"=w52:dbl, "Not In Sight?"=w47:bool, "In Range?"=w48:bool)  [unwired: 8 in]
          n33 = case shown="True" w47 {
            selector: w47 -> [_ w69]
            tunnel: w53 -> [w55 _]
            tunnel: w52 -> [w54 _]
            frame False {
              n34 = call <vilib>:"WPI_MotorControlRefNum Registry Get.vi"("refnum name"="Drive R0") -> ("error out"=w61:errorcluster, "MotorControlDevRef"=w57:T5)  [unwired: 9 in]
              n35 = call <vilib>:"WPI_MotorControlRefNum Registry Get.vi"("refnum name"="Drive R1") -> ("error out"=w56:errorcluster, "MotorControlDevRef"=w59:T5)  [unwired: 9 in]
              n36 = call <vilib>:"WPI_MotorControlRefNum Registry Get.vi"("refnum name"="Drive L0") -> ("error out"=w62:errorcluster, "MotorControlDevRef"=w63:T5)  [unwired: 9 in]
              n37 = call <vilib>:"WPI_MotorControlRefNum Registry Get.vi"("refnum name"="Drive L1") -> ("error out"=w66:errorcluster, "MotorControlDevRef"=w65:T5)  [unwired: 9 in]
              n38 = call <vilib>:"WPI_MotorControlSetOutput.vi"("error in (no error)"=w61, "Output"=w55, "MotorControlDevRef"=w57) -> ()  [unwired: 6 in, 3 out]
              n39 = call <vilib>:"WPI_MotorControlSetOutput.vi"("error in (no error)"=w56, "Output"=w55, "MotorControlDevRef"=w59) -> ()  [unwired: 6 in, 3 out]
              n40 = call <vilib>:"WPI_MotorControlSetOutput.vi"("error in (no error)"=w62, "Output"=w54, "MotorControlDevRef"=w63) -> ()  [unwired: 6 in, 3 out]
              n41 = call <vilib>:"WPI_MotorControlSetOutput.vi"("error in (no error)"=w66, "Output"=w54, "MotorControlDevRef"=w65) -> ()  [unwired: 6 in, 3 out]
            }
            frame True {
              n42 = Not(x=w69) -> (.not. x?=w68:bool)
              n43 = call "Oscillate.vi"("Target In Sight?"=w68, "Effort"=0.25) -> ()  [unwired: 10 in]
            }
          }
        }
      }
      frame "Turn", Default {
        n44 = flat-sequence {
          tunnel: w73 -> [w77]
          tunnel: w72 -> [w76]
          tunnel: w71 -> [w74]
          frame #0 {
            n45 = To Long Integer(number=w74) -> (32bit integer=w75:i32)
            n46 = Wait (ms)(milliseconds to wait=w76) -> ()  [unwired: 1 out]
            n47 = call "Turn.vi"("mode"=w75, "Effort"=w77) -> ()  [unwired: 10 in]
          }
          frame #1 {
            n48 = call "Turn.vi"("mode"=1, "Effort"=0.0) -> ()  [unwired: 10 in]
          }
        }
      }
      frame "Intake" {
        n49 = flat-sequence {
          tunnel: w81 -> [w83]
          tunnel: w80 -> [w82]
          frame #0 {
            n50 = Wait (ms)(milliseconds to wait=w82) -> ()  [unwired: 1 out]
            n51 = call "Intake.vi"("Effort"=w83) -> ()  [unwired: 11 in]
          }
          frame #1 {
            n52 = call "Intake.vi"("Effort"=0.0) -> ()  [unwired: 11 in]
          }
        }
      }
      frame "Test" {
      }
      frame "Gear0" {
        n53 = flat-sequence {
          tunnel: w85 -> [w89]
          frame #0 {
            n54 = To Unsigned Byte Integer(number=w89) -> (unsigned 8bit integer=w88:u8)
            n55 = Number To Boolean Array(number=w88) -> (Boolean array=w87:bool[])
            n56 = Index Array(array=w87) -> (element=w86:bool)  [unwired: 1 in]
            n57 = call "Gear.vi"("Gear0?"=w86) -> ()  [unwired: 11 in]
          }
        }
      }
      frame "Gear1" {
        n58 = flat-sequence {
          tunnel: w90 -> [w94]
          frame #0 {
            n59 = To Unsigned Byte Integer(number=w94) -> (unsigned 8bit integer=w93:u8)
            n60 = Number To Boolean Array(number=w93) -> (Boolean array=w92:bool[])
            n61 = Index Array(array=w92) -> (element=w91:bool)  [unwired: 1 in]
            n62 = call "Gear.vi"("Gear1?"=w91) -> ()  [unwired: 11 in]
          }
        }
      }
      frame "Index" {
        n63 = flat-sequence {
          tunnel: w96 -> [w97]
          tunnel: w95 -> [_]
          frame #0 {
            n64 = Wait (ms)(milliseconds to wait=w97) -> ()  [unwired: 1 out]
            n65 = call "Index.vi"("millisecond timer value"=w97, "Shoot"=TRUE ("Override?"), "Output"=-1.0) -> ()  [unwired: 9 in]
          }
          frame #1 {
            n66 = call "Index.vi"("Shoot"=FALSE ("Override?"), "Output"=0.0) -> ()  [unwired: 10 in]
          }
        }
      }
      frame "Climb" {
        n67 = flat-sequence {
          tunnel: w103 -> [w105]
          tunnel: w102 -> [w104]
          frame #0 {
            n68 = call "Climb.vi"("Effort"=w105) -> ()  [unwired: 11 in]
            n69 = Wait (ms)(milliseconds to wait=w104) -> ()  [unwired: 1 out]
          }
          frame #1 {
            n70 = call "Climb.vi"("Effort"=0.0) -> ()  [unwired: 11 in]
          }
        }
      }
      frame "Drive Encoder Reset" {
        n71 = while {
          stop <- w107 stop-if-true
          n72 = call <vilib>:"WPI_MotorControlRefNum Registry Get.vi"("refnum name"="Drive L1") -> ("error out"=w117:errorcluster, "MotorControlDevRef"=w112:T5)  [unwired: 9 in]
          n73 = call <vilib>:"WPI_MotorControlRefNum Registry Get.vi"("refnum name"="Drive R1") -> ("error out"=w122:errorcluster, "MotorControlDevRef"=w121:T5)  [unwired: 9 in]
          n74 = call <vilib>:"WPI_MotorControlRefNum Registry Get.vi"("refnum name"="Drive L1") -> ("error out"=w124:errorcluster, "MotorControlDevRef"=w125:T5)  [unwired: 9 in]
          n75 = call <vilib>:"WPI_MotorControlRefNum Registry Get.vi"("refnum name"="Drive R1") -> ("error out"=w114:errorcluster, "MotorControlDevRef"=w113:T5)  [unwired: 9 in]
          n76 = call <vilib>:"WPI_CANTalonSRX_SetSensorPosition.vi"("error in (no error)"=w122, "New Sensor Position"=0.0, "CAN Talon SRX Ref"=w121) -> ()  [unwired: 7 in, 2 out]
          n77 = call <vilib>:"WPI_CANTalonSRX_SetSensorPosition.vi"("error in (no error)"=w124, "New Sensor Position"=0.0, "CAN Talon SRX Ref"=w125) -> ()  [unwired: 7 in, 2 out]
          n78 = call <vilib>:"WPI_CANTalonSRX_GetStatus.vi"("error in (no error)"=w117, "CAN Talon SRX Ref"=w112) -> ("Talon SRX Status"=w115:T9)  [unwired: 7 in, 2 out]
          n79 = Unbundle By Name(w115) -> ("Encoder Position"=w110:dbl)
          n80 = call <vilib>:"WPI_CANTalonSRX_GetStatus.vi"("error in (no error)"=w114, "CAN Talon SRX Ref"=w113) -> ("Talon SRX Status"=w116:T9)  [unwired: 7 in, 2 out]
          n81 = Unbundle By Name(w116) -> ("Encoder Position"=w111:dbl)
          n82 = Equal To 0?(x=w110) -> (x = 0?=w109:bool)
          n83 = Equal To 0?(x=w111) -> (x = 0?=w108:bool)
          n84 = And(x=w109, y=w108) -> (x .and. y?=w107:bool)
        }
      }
      frame "Gyro Reset" {
        n85 = call <vilib>:"WPI_GyroRefNum Registry Get.vi"("refnum name"="Gyro") -> ("error out"=w129:errorcluster, "GyroDevRef"=w130:T10)  [unwired: 9 in]
        n86 = call <vilib>:"WPI_GyroReset.vi"("error in"=w129, "GyroDevRef"=w130) -> ()  [unwired: 8 in, 2 out]
      }
    }
  }
